vi "Convert Detection Robot to AI Robot.vi"(5 "fps":dbl, 7 "Lado":enum16{"Esquerdo", "Direito"}(ring) caption="Enum", 11 "Input":T6[](array[typedef]) {"height" format="%+4.3f"; "pixel_y" format="%+4.3f"; "pixel_x" format="%+4.3f"; "orientation" format="%+4.3f"; "y" format="%+4.3f"; "confidence" format="%4.3f"; "x" format="%+4.3f"}) -> (3 "Output":T1[](array[typedef]))   [LabVIEW 2018]
uses:
  SSL Detection Robot.ctl
  <vilib>/Analysis/Matrix/Datatypes/RealMatrix.ctl
  AI Robot.ctl
  Intel/Functions Enum.ctl
  Intel/AttackerStates.ctl
  Path Planning/RRT/PathDests.ctl
  Path Planning/RRT/PathDest.ctl
  <vilib>/Analysis/Matrix/NI_Matrix.lvlib
panel:
  in  "fc":dbl=15.0
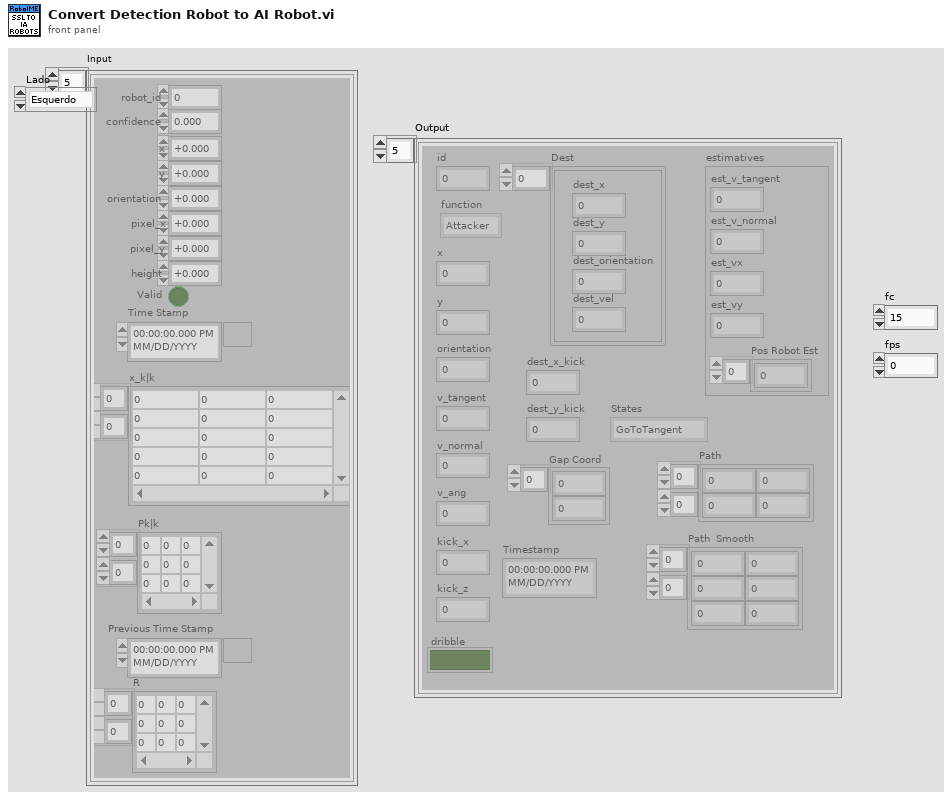
[diagram p1: front panel]
types:
  T1 = typedef "AI Robot.ctl" = cluster{"id":u32, "function":T2, "x":dbl, "y":dbl, "orientation":dbl, "v_tangent":dbl, "v_normal":dbl, "v_ang":dbl, "kick_x":dbl, "kick_z":dbl, "dribble":bool, "Timestamp":timestamp, "estimatives":cluster{"est_v_tangent":dbl, "est_v_normal":dbl, "est_vx":dbl, "est_vy":dbl, "Pos Robot Est":dbl[]}, "dest_x_kick":dbl, "dest_y_kick":dbl, "Gap Coord":dbl[], "States":T3, "Path ":dbl[][], "Path  Smooth":dbl[][], "Dest":T4}
  T2 = typedef "Functions Enum.ctl" = enum16{"2nd Striker", "Attacker", "Goalie", "Defender", "Striker", "Goto 0", "Dummy", "Kicker", "ZigZag 0", "ZigZag 1", "ZigZag 2", "ZigZag 3", "ZigZag 4", "ZigZag 5", "ZigZag 6", "ZigZag 7", "ZigZag 8", ""}
  T3 = typedef "AttackerStates.ctl" = enum16{"Pass", "GoToTangent", "BallGetting", "GoToKick", ""}
  T4 = typedef "PathDests.ctl" = T5[]
  T5 = typedef "PathDest.ctl" = cluster{"dest_x":dbl, "dest_y":dbl, "dest_orientation":dbl, "dest_vel":dbl}
  T6 = typedef "SSL Detection Robot.ctl" = cluster{"x":sgl, "robot_id":u32, "confidence":sgl, "y":sgl, "orientation":sgl, "pixel_x":sgl, "pixel_y":sgl, "height":sgl, "Valid":bool, "Time Stamp":timestamp, "x_k|k":T7, "Pk|k":T7, "Previous Time Stamp":timestamp, "R":T7}
  T7 = typedef "NI_Matrix.lvlib/RealMatrix.ctl" = dbl[][]
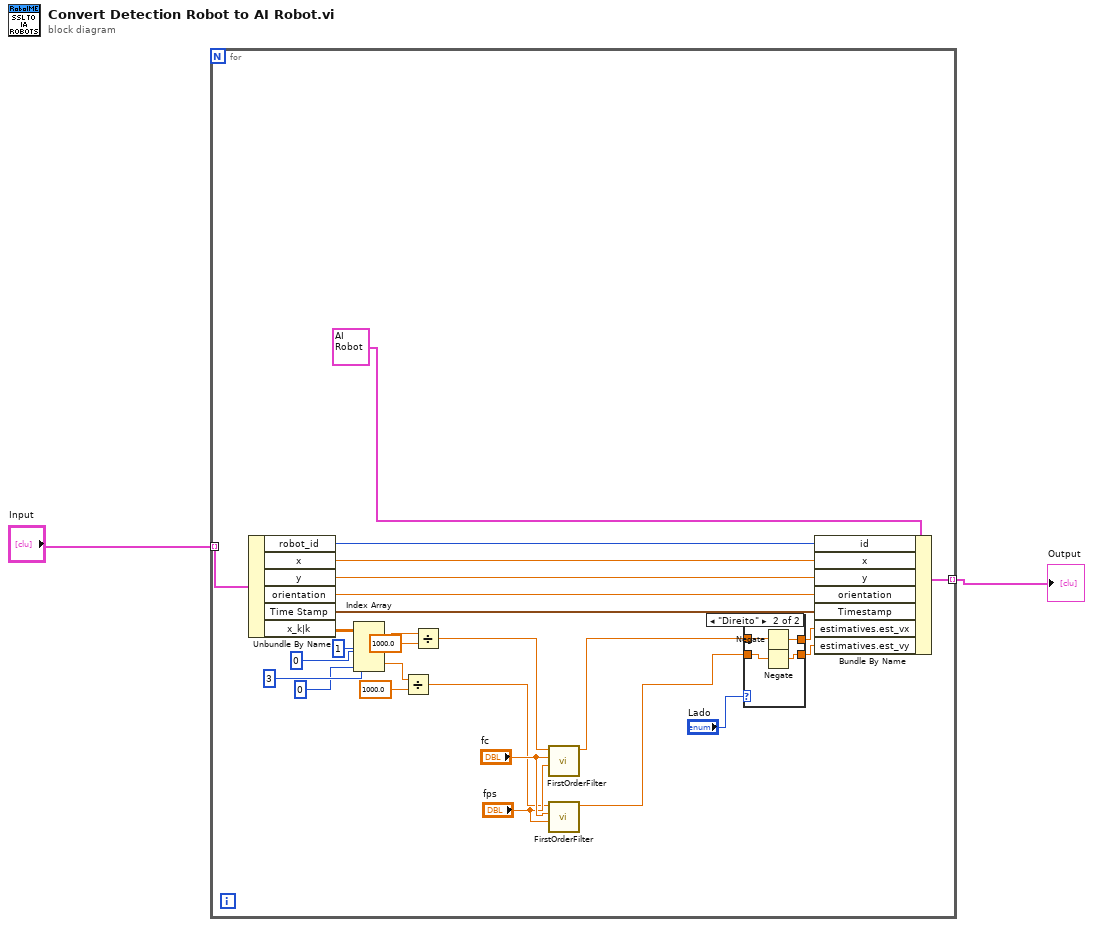
[diagram p0: block diagram]
diagram:
  n1 = for {
    tunnel: "Input" -> [w27] mode=indexing
    tunnel: [w21] -> w1 mode=indexing
    n2 = Unbundle By Name(w27) -> ("robot_id"=w26:u32, "x"=w25:sgl, "y"=w24:sgl, "orientation"=w23:sgl, "Time Stamp"=w22:timestamp, "x_k|k"=w20:T7)
    n3 = Index Array(array=w20, index (row) #1=1 ("index (row)"), index (col) #1=0 ("disabled index (col)"), index (row) #2=3 ("index (row)"), index (col) #2=0 ("disabled index (col)")) -> (element #1=w15:dbl, element #2=w12:dbl)
    n4 = Divide(x=w12, y=1000.0) -> (x/y=w4:dbl)
    n5 = Divide(x=w15, y=1000.0) -> (x/y=w6:dbl)
    n6 = call "FirstOrderFilter.vi"("fps"="fps", "fc"="fc", "Numeric in"=w6) -> ("Numeric out"=w5:dbl)  [unwired: 8 in]
    n7 = call "FirstOrderFilter.vi"("fps"="fps", "fc"="fc", "Numeric in"=w4) -> ("Numeric out"=w3:dbl)  [unwired: 8 in]
    n8 = case shown="\"Direito\"" "Lado" {
      tunnel: [w30 w34] -> w10
      tunnel: w5 -> [w30 w33]
      tunnel: [w29 w31] -> w9
      tunnel: w3 -> [w29 w32]
      frame "Esquerdo", Default {
      }
      frame "Direito" {
        n9 = Negate(x=w33) -> (-x=w34:dbl)
        n10 = Negate(x=w32) -> (-x=w31:dbl)
      }
    }
    n11 = Bundle By Name(cluster=T1 {"id"=0, "function"=enum."Attacker", "x"=0.0, "y"=0.0, "orientation"=0.0, "v_tangent"=0.0, "v_normal"=0.0, "v_ang"=0.0, "kick_x"=0.0, "kick_z"=0.0, "dribble"=FALSE, "Timestamp"=timestamp(0 s since 1904-01-01), "estimatives"={"est_v_tangent"=0.0, "est_v_normal"=0.0, "est_vx"=0.0, "est_vy"=0.0, "Pos Robot Est"=[]}, "dest_x_kick"=0.0, "dest_y_kick"=0.0, "Gap Coord"=[], "States"=enum."GoToTangent", "Path "=[], "Path  Smooth"=[], "Dest"=[]} ("Robot"), "id"=w26, "x"=w25, "y"=w24, "orientation"=w23, "Timestamp"=w22, "estimatives.est_vx"=w10, "estimatives.est_vy"=w9) -> (w21:T1)
  }
  "Output" <- w1
